vi "Set Bit.vi"(9 "bit value":bool, 10 "bit index":u8, 11 "value in":u8 format="%08b") -> (3 "value out":u8 format="%08b")   [LabVIEW 2017, in "DSF Core.lvlib" / "Buffer Converter.lvclass"]
uses:
  Buffer Converter.lvclass
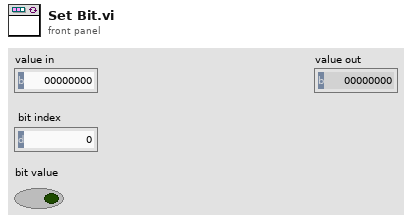
[diagram p1: front panel]
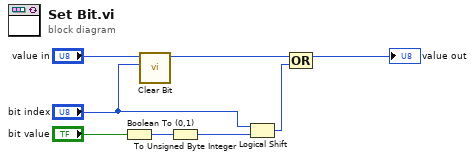
[diagram p0: block diagram]
diagram:
  n1 = Boolean To (0,1)(Boolean="bit value") -> (0, 1=w6:i16)
  n2 = call "Clear Bit.vi"("bit index"="bit index", "value in"="value in") -> ("value out"=w2:u8)  [unwired: 9 in]
  n3 = To Unsigned Byte Integer(number=w6) -> (unsigned 8bit integer=w5:u8)
  n4 = Logical Shift(y="bit index", x=w5) -> (x << y=w3:u8)
  n5 = Compound Arithmetic op=OR(w2, w3) -> (→"value out":u8)
